vi "Create Electrode Array.vi"(8 "Insert\nBreak":bool=TRUE, 9 "Inverse\nPolarity":bool=TRUE, 10 "Electrode number, N":u16=100, 11 "Array Mode":u16(ring) items=["None", "Gradient + Dipole dipole", "Gradient", "Dipole Dipole", "Schlumberger"]) -> (3 "Current Mode":u8[][](array[numeric]))   [LabVIEW 2023]
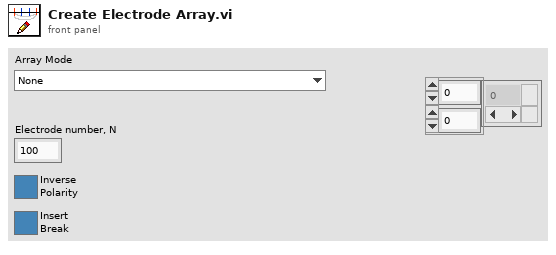
[diagram p1: front panel]
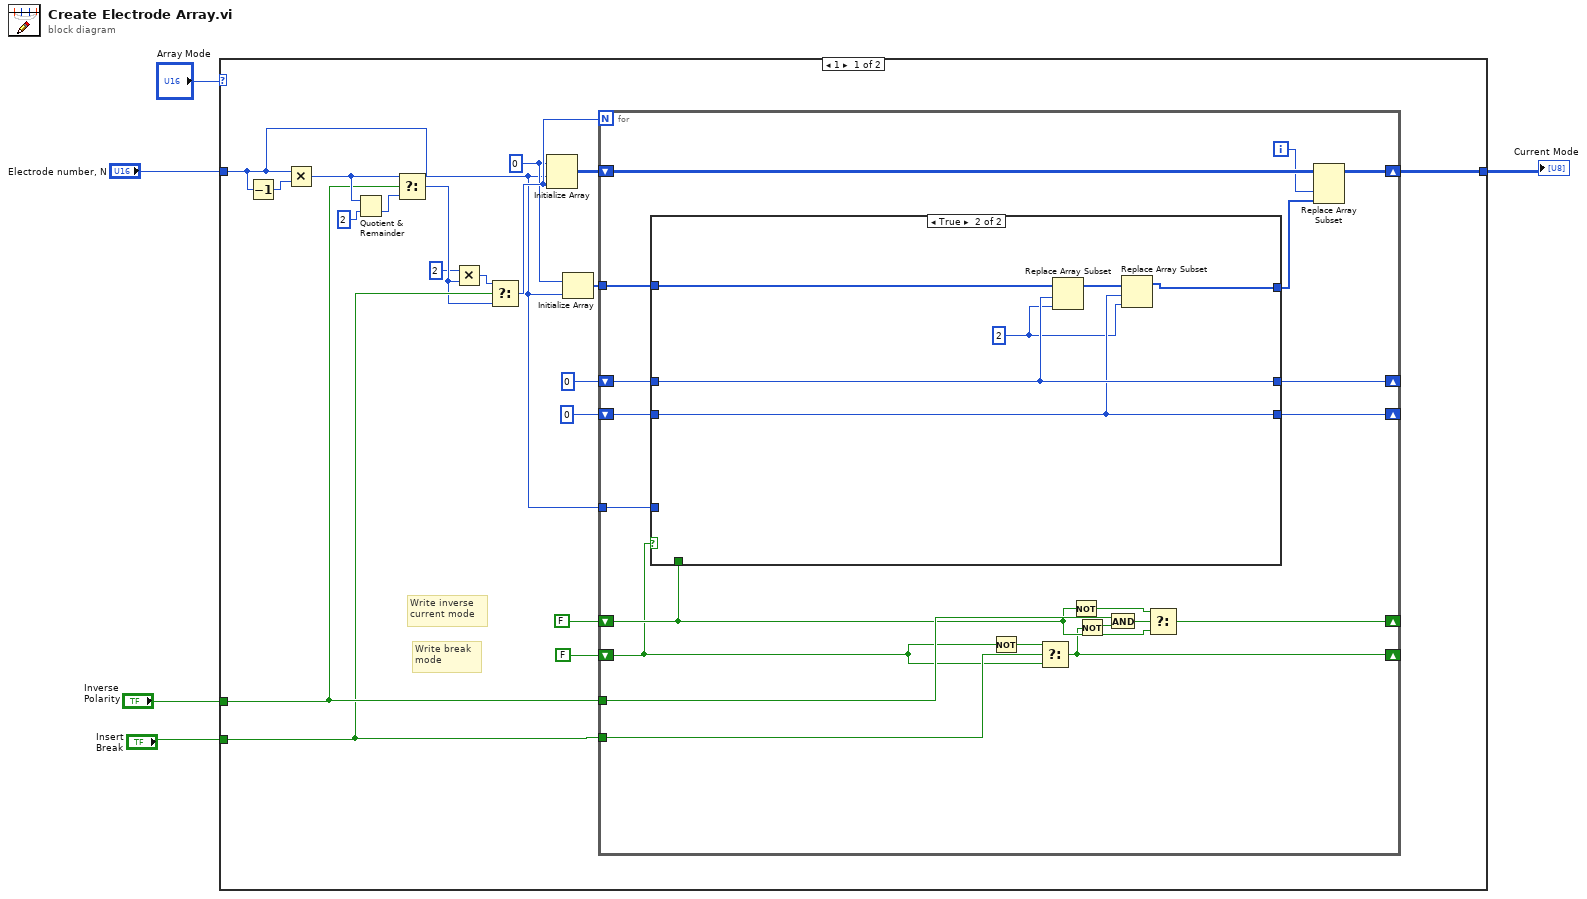
[diagram p0: block diagram]
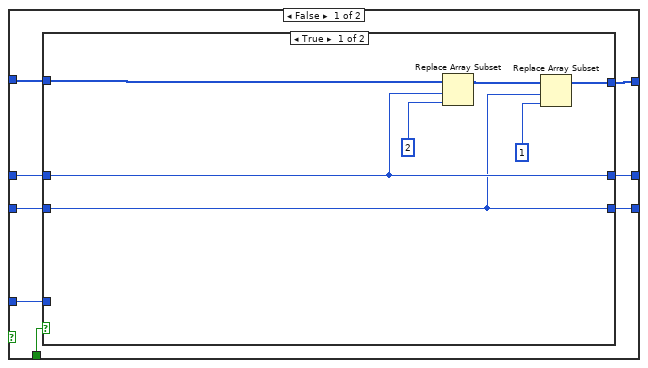
[diagram p2: hidden frame]
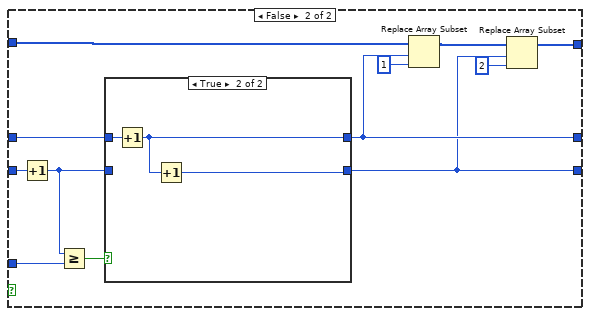
[diagram p3: hidden frame]
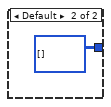
[diagram p5: hidden frame]
diagram:
  n1 = case shown="1" "Array Mode" {
    tunnel: "Electrode number, N" -> [w9 _]
    tunnel: "Inverse\nPolarity" -> [w14 _]
    tunnel: "Insert\nBreak" -> [w13 _]
    tunnel: [w10 u8[][] []] -> w1
    frame 1 {
      w11 = u8 0 ("stateArray")
      # "Write break\nmode"
      # "Write inverse\ncurrent mode"
      n2 = Decrement(x=w9) -> (x-1=w24:u16)
      n3 = Multiply(x=w9, y=w24) -> (x*y=w23:u16)
      n4 = Quotient & Remainder(x=w23, y=u16 2) -> (floor(x/y)=w21:u16)  [unwired: 1 out]
      n5 = Select(t=w23, s=w14, f=w21) -> (s? t:f=w7:u16)
      n6 = Multiply(x=u16 2, y=w7) -> (x*y=w8:u16)
      n7 = Select(t=w8, s=w13, f=w7) -> (s? t:f=w19:u16)
      n8 = Initialize Array(w11, w9, w19) -> (w20:u8[][])
      n9 = Initialize Array(w11, w9) -> (w12:u8[])
      n10 = for {
        N: w19 -> [_]
        shift-right: [w29] -> w10
        shift-left: w20 -> [w44]
        shift-right: [w32] -> _
        shift-left: 0 ("index (row)") -> [w35]
        shift-right: [w31] -> _
        shift-left: 0 ("index (row)") -> [w34]
        shift-right: [w39] -> _
        shift-left: FALSE ("Insert\nBreak") -> [w36]
        shift-right: [w26] -> _
        shift-left: FALSE ("Insert\nBreak") -> [w27]
        tunnel: w14 -> [w43]
        tunnel: w13 -> [w42]
        tunnel: w12 -> [w37]
        tunnel: w9 -> [w33]
        i -> [w38]
        n11 = case shown="True" w27 {
          tunnel: w37 -> [w51 w82]
          tunnel: [w48 w77] -> w30
          tunnel: w36 -> [w52 _]
          tunnel: w35 -> [w50 w81]
          tunnel: w34 -> [w49 w79]
          tunnel: w33 -> [w47 _]
          tunnel: [w46 w81] -> w32
          tunnel: [w45 w79] -> w31
          frame False {
            n12 = case shown="True" w52 {
              tunnel: w51 -> [w59 w71]
              tunnel: w50 -> [w54 w63]
              tunnel: w49 -> [w53 w66]
              tunnel: [w55 w67] -> w48
              tunnel: w47 -> [_ w65]
              tunnel: [w54 w61] -> w46
              tunnel: [w53 w60] -> w45
              frame True {
                n13 = Replace Array Subset(array=w59, new element=u8 2 ("new element/subarray"), index=w54) -> (w56:u8[])
                n14 = Replace Array Subset(array=w56, new element=u8 1 ("new element/subarray"), index=w53) -> (w55:u8[])
              }
              frame False {
                n15 = Increment(x=w66) -> (x+1=w62:i32)
                n16 = Greater Or Equal?(x=w62, y=w65) -> (x >= y?=w64:bool)
                n17 = case shown="True" w64 {
                  tunnel: w63 -> [w72 w76]
                  tunnel: [w72 w75] -> w61
                  tunnel: [w73 w74] -> w60
                  tunnel: w62 -> [w73 _]
                  frame False {
                  }
                  frame True {
                    n18 = Increment(x=w76) -> (x+1=w75:i32)
                    n19 = Increment(x=w75) -> (x+1=w74:i32)
                  }
                }
                n20 = Replace Array Subset(array=w71, new element=u8 1 ("new element/subarray"), index=w61) -> (w68:u8[])
                n21 = Replace Array Subset(array=w68, new element=u8 2 ("new element/subarray"), index=w60) -> (w67:u8[])
              }
            }
          }
          frame True {
            w78 = u8 2 ("new element/subarray")
            n22 = Replace Array Subset(array=w82, new element=w78, index=w81) -> (w80:u8[])
            n23 = Replace Array Subset(array=w80, new element=w78, index=w79) -> (w77:u8[])
          }
        }
        n24 = Not(x=w27) -> (.not. x?=w41:bool)
        n25 = Select(t=w41, s=w42, f=w27) -> (s? t:f=w26:bool)
        n26 = Not(x=w36) -> (.not. x?=w40:bool)
        n27 = Not(x=w26) -> (.not. x?=w25:bool)
        n28 = And(x=w43, y=w25) -> (x .and. y?=w28:bool)
        n29 = Select(t=w40, s=w28, f=w36) -> (s? t:f=w39:bool)
        n30 = Replace Array Subset(array=w44, new element=w30, index (col)=w38) -> (w29:u8[][])  [unwired: 1 in]
      }
    }
    frame Default {
    }
  }
  "Current Mode" <- w1
